vi "S2DS_User list (SubVI).vi"(8 "error in (no error)":errorcluster) -> (0 "error out":errorcluster, 1 "Current user":string, 2 "User list":string[](array[string]), 3 "File index":u32)   [LabVIEW 2025]
uses:
  <vilib>/Utility/config.llb/Read Key (I32).vi
  <vilib>/Utility/config.llb/Read Key (String).vi
  <vilib>/Utility/config.llb/Read Key (U32).vi
  <vilib>/Utility/config.llb/NI_LVConfig.lvlib
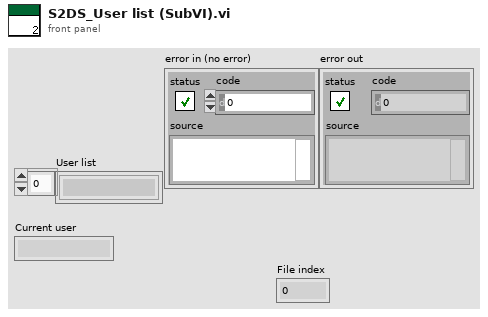
[diagram p1: front panel]
types:
  T1 = typedef "NI_LVConfig.lvlib/Config Data RefNum.ctl" = refnum<k1>
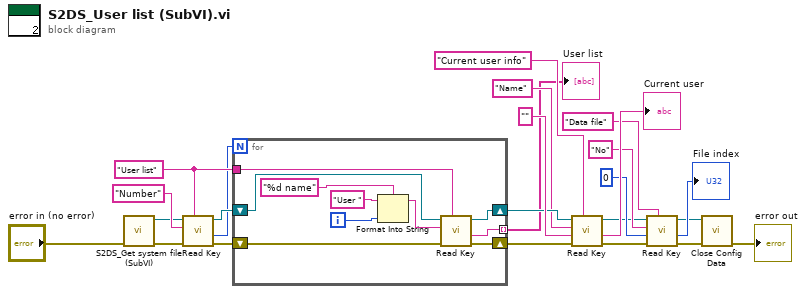
[diagram p0: block diagram]
diagram:
  w17 = "User list" ("section")
  n1 = call "S2DS_Get system file (SubVI).vi"("error in (no error)"="error in (no error)") -> ("error out"=w11:errorcluster, "Refnum out"=w12:T1)  [unwired: 9 in]
  n2 = call-poly <vilib>:"Read Key.vi"("section"=w17, "error in (no error)"=w11, "key"="Number", "refnum"=w12) -> ("error out"=w16:errorcluster, "value"=w14:i32, "refnum out"=w15:T1)  [unwired: 4 in, 1 out]
  n3 = for {
    N: w14 -> [_]
    shift-right: [w33] -> w20
    shift-left: w15 -> [w34]
    shift-right: [w31] -> w22
    shift-left: w16 -> [w32]
    tunnel: w17 -> [w30]
    tunnel: [w25] -> w18 mode=indexing
    i -> [w27]
    n4 = Format Into String(format string="%d name", initial string="User " ("key"), w27) -> (resulting string=w26:string)  [unwired: 1 in, 1 out]
    n5 = call-poly <vilib>:"Read Key.vi"("section"=w30, "error in (no error)"=w32, "key"=w26, "refnum"=w34) -> ("error out"=w31:errorcluster, "value"=w25:string, "refnum out"=w33:T1)  [unwired: 4 in, 1 out]
  }
  "User list" <- w18
  n6 = call-poly <vilib>:"Read Key.vi"("section"="Current user info", "error in (no error)"=w22, "default value"="", "key"="Name", "refnum"=w20) -> ("error out"=w2:errorcluster, "value"=→"Current user":string, "refnum out"=w4:T1)  [unwired: 3 in, 1 out]
  n7 = call-poly <vilib>:"Read Key.vi"("section"="Data file", "error in (no error)"=w2, "default value"=u32 0, "key"="No", "refnum"=w4) -> ("error out"=w1:errorcluster, "value"=→"File index":u32, "refnum out"=w3:T1)  [unwired: 3 in, 1 out]
  n8 = call <vilib>:"Close Config Data.vi"("error in (no error)"=w1, "refnum"=w3) -> ("error out"=→"error out":errorcluster)  [unwired: 8 in, 1 out]
